vi "GetSequenceFullName.vi"(8 "error in":errorcluster, 11 "SequenceRun in":refnum<class "SequenceRun.lvclass">) -> (0 "error out":errorcluster, 2 "SequenceFullName":string, 3 "SequenceRun out":refnum<class "SequenceRun.lvclass">)   [LabVIEW 2021, in "ProligentXMLGenerator.lvlib" / "SequenceRun.lvclass"]
doc: "Defines the full name of the sequence executed in this sequence run.\n\"[Root Sequence/][[Path/]...]SequenceName\"\nEach path strings and the sequence name are limited to 264 characters and the total string provided is limited to 2000 characters\n\nWARNING:\n\nSince the '/' character is the hierarchy delimiter, if a path string contains a '/' character it will be interpreted as\na new hierarchy. It is therefore suggested to replace '/' by '-' in all your path components to keep the expected hierarchy.\nFor example, if you have a sequence named 'PASS/FAIL' and you don't substitude '/' by '-', the 'PASS' would be interpreted\nas a sequence category while 'FAIL' would be the name of a sequence. If you do the suggested substitution, the name of\nthe sequence would be interpreted as 'PASS-FAIL' without any category."
uses:
  SequenceRun.lvclass
  SequenceRun.lvclass/SequenceRun.ctl
  Base/SequenceFullName/SequenceFullName.lvclass
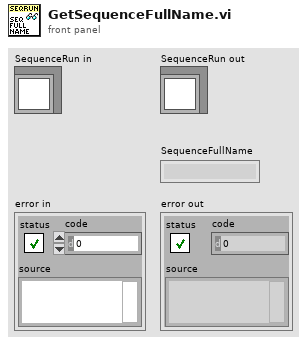
[diagram p1: front panel]
types:
  T1 = typedef "ProligentXMLGenerator.lvlib/SequenceRun.lvclass/Data.ctl" = cluster{"Name":string, "StepRuns":refnum<class "StepRun.lvclass">[], "Characteristics":refnum<class "Characteristic.lvclass">[], "Documents":refnum<class "Document.lvclass">[], "FailureReferences":refnum<class "FailureReference.lvclass">[], "CustomData":refnum<class "CustomData.lvclass">, "StartDate":refnum<class "DateTime.lvclass">, "EndDate":refnum<class "DateTime.lvclass">, "SequenceExecutionStatus":refnum<class "ExecutionStatus.lvclass">, "SequenceRunId":refnum<class "Guid.lvclass">, "SequenceFullName":refnum<class "SequenceFullName.lvclass">, "SequenceVersion":refnum<class "NonEmptyString_64.lvclass">, "StationFullName":refnum<class "FullName.lvclass">, "User":refnum<class "NonEmptyString_255.lvclass">, "TimeZoneInfoId":string}
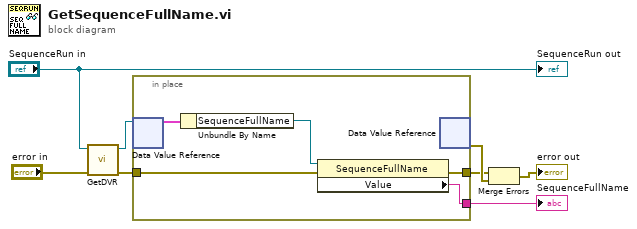
[diagram p0: block diagram]
diagram:
  n1 = call "GetDVR.vi"("error in"="error in", "SequenceRun"="SequenceRun in") -> ("error out"=w2:errorcluster, "DVRReference"=w7:refnum<data-value>)  [unwired: 8 in]
  n2 = in-place "In Place Element Structure" {
    in-place-border: [w10] -> w6
    in-place-border: w2 -> [w11]
    in-place-border: [w9] -> w1
    n3 = in-place-dvr #1(w7) -> (w13:T1)  [unwired: 1 out]
    n4 = Unbundle By Name(w13) -> ("SequenceFullName"=w12:refnum<class "SequenceFullName.lvclass">)
    n5 = property on="Property Node" class="SequenceFullName"(reference=w12, error in=w11) -> (error out=w9:errorcluster, "Value"=w10:string)  [unwired: 1 out]
    n6 = in-place-dvr #1() -> (w8:errorcluster)  [unwired: 1 in, 1 out]
  }
  "SequenceFullName" <- w6
  n7 = Merge Errors(w1, w8) -> (→"error out":errorcluster)
  "SequenceRun out" <- "SequenceRun in"
